vi "Get PNG Chunks.vi"(11 "data":string) -> (0 "CRC":string[](array[string]), 1 "Data":string[](array[string]), 2 "Name":string[](array[string]), 3 "Length":u32[](array[numeric]), 4 "Chunks":string[](array[string]), 5 "Header":string)   [LabVIEW 2009]
doc: "Retrieves all chunks from a PNG file.\nCreated by Darin"
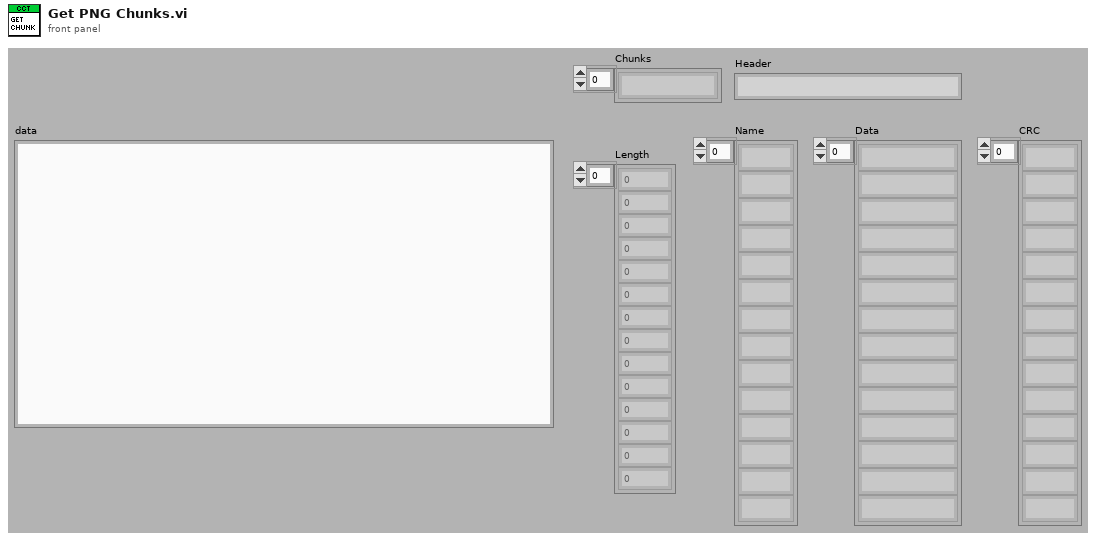
[diagram p1: front panel]
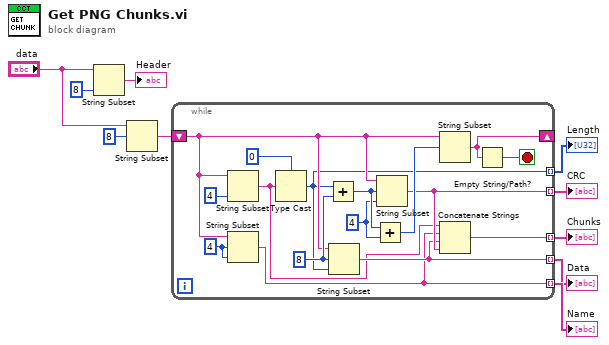
[diagram p0: block diagram]
diagram:
  n1 = String Subset(string="data", length (rest)=8 ("length (rest)")) -> (substring=→"Header":string)  [unwired: 1 in]
  n2 = String Subset(string="data", offset (0)=8 ("length (rest)")) -> (substring=w1:string)  [unwired: 1 in]
  n3 = while {
    shift-right: [w16] -> _
    shift-left: w1 -> [w19]
    tunnel: [w17] -> w10 mode=indexing
    tunnel: [w14] -> w8 mode=indexing
    tunnel: [w15] -> w7 mode=indexing
    tunnel: [w13] -> w9 mode=indexing
    tunnel: [w11] -> w6 mode=indexing
    stop <- w18 stop-if-true
    w20 = 4 ("length (rest)")
    w23 = 8 ("offset (0)")
    w24 = 4 ("length (rest)")
    n4 = String Subset(string=w19, length (rest)=4 ("length (rest)")) -> (substring=w12:string)  [unwired: 1 in]
    n5 = String Subset(string=w19, offset (0)=w24, length (rest)=w24) -> (substring=w13:string)
    n6 = Type Cast(type=u32 0, x=w12) -> (*(type *) &x=w17:u32)
    n7 = Add(x=w17, y=w23) -> (x+y=w21:u32)
    n8 = String Subset(string=w19, offset (0)=w23, length (rest)=w17) -> (substring=w14:string)
    n9 = Add(x=w21, y=w20) -> (x+y=w22:u32)
    n10 = String Subset(string=w19, offset (0)=w21, length (rest)=w20) -> (substring=w15:string)
    n11 = String Subset(string=w19, offset (0)=w22) -> (substring=w16:string)  [unwired: 1 in]
    n12 = Concatenate Strings(w12, w13, w14, w15) -> (w11:string)
    n13 = Empty String/Path?(string/path=w16) -> (empty?=w18:bool)
  }
  "Length" <- w10
  "Name" <- w9
  "Data" <- w8
  "CRC" <- w7
  "Chunks" <- w6
